vi "Set Magnet Vector Field.vi"(8 "error in (no error)":errorcluster, 9 "Target Rate (T/min)":dbl, 10 "Target Field (T)":dbl[](array[numeric]), 11 "Instrument.VRM in":refnum<class "Instrument.OxfordVRM.lvclass">) -> (0 "error out":errorcluster, 3 "Instrument.VRM out":refnum<class "Instrument.OxfordVRM.lvclass">)   [LabVIEW 2019, in "Instrument.OxfordVRM.lvclass"]
uses:
  Instrument.OxfordVRM.lvclass
  Typedefs/Instrument.VRM.Commands-enum.ctl
  Typedefs/Instrument.VRM.setMagnet-cluster.ctl
  Typedefs/VRM Targets--Cluster.ctl
  Typedefs/VRM Magnet Axis--Enum.ctl
  5e873d59-b7fa-4b76-b36a-7150f831c1b5.vi
  5e873d59-b7fa-4b76-b36a-7150f831c1b5.vi/9026e099-2f45-42fd-b5f2-7045f12962a4.vi
  5e873d59-b7fa-4b76-b36a-7150f831c1b5.vi/9026e099-2f45-42fd-b5f2-7045f12962a4.vi/94005640-8c22-463d-97a2-e8991734048f.vi
  5e873d59-b7fa-4b76-b36a-7150f831c1b5.vi/9026e099-2f45-42fd-b5f2-7045f12962a4.vi/52164787-c95e-474d-af3d-433121107a3c.vi
  5e873d59-b7fa-4b76-b36a-7150f831c1b5.vi/9026e099-2f45-42fd-b5f2-7045f12962a4.vi/52164787-c95e-474d-af3d-433121107a3c.vi/53ccfac9-2453-43af-8059-1cd8c477cd5d.vi
  <userlib>/LevyLab/Levylab Instruments/SMOs/RemoteControl/API/Remote Client.vi
  <vilib>/JDP Science/JSONtext/JSON text to Variant.vi
  <vilib>/JDP Science/JSONtext/LVClass Serializer/JSONtext LVClass Serializer.lvclass
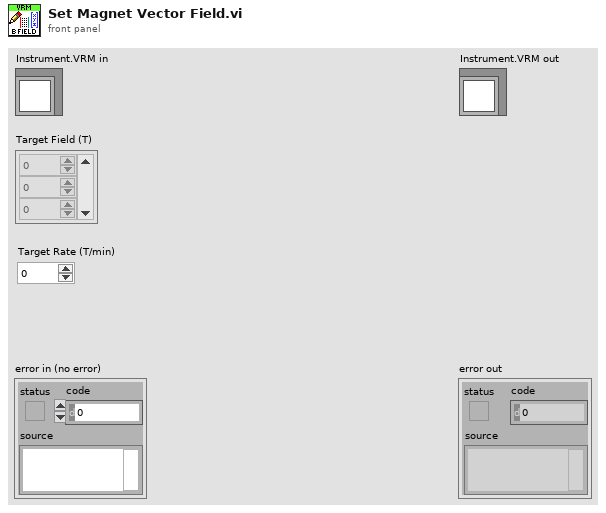
[diagram p1: front panel]
types:
  T1 = typedef "Instrument.OxfordVRM.lvclass/VRM Magnet Axis--Enum.ctl" = enum16{"Z", "X", "Y", "ALL"}
  T2 = typedef "Instrument.OxfordVRM.lvclass/Instrument.VRM.setMagnet-cluster.ctl" = cluster{"Target":T3}
  T3 = typedef "Instrument.OxfordVRM.lvclass/VRM Targets--Cluster.ctl" = cluster{"Field (T)":dbl[], "Field Rate (T/min)":dbl, "Axis":T1}
  T4 = typedef "Instrument.OxfordVRM.lvclass/Instrument.VRM.Commands-enum.ctl" = enum16{"setAction", "setTarget", "setMagnetField", "getStatus", "getTarget", "getMagnetField"}
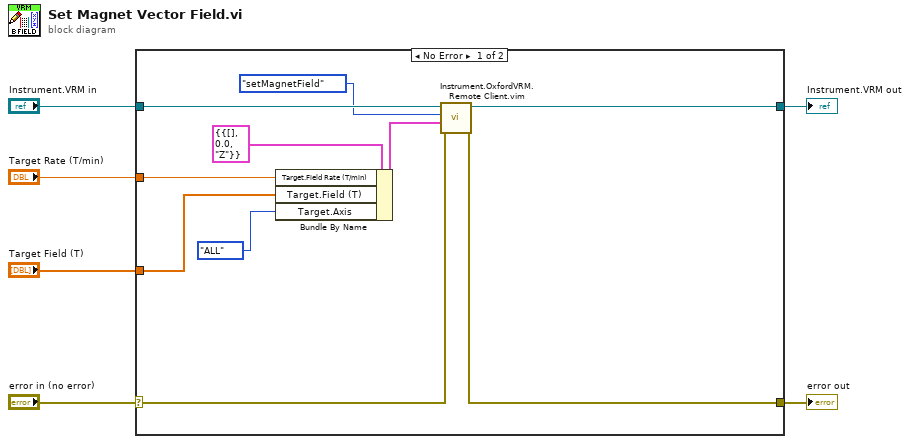
[diagram p0: block diagram]
diagram:
  n1 = case shown="No Error" "error in (no error)" {
    selector: "error in (no error)" -> [w12 w18]
    tunnel: [w8 w18] -> w6
    tunnel: "Instrument.VRM in" -> [w16 w17]
    tunnel: [w15 w17] -> w4
    tunnel: "Target Field (T)" -> [w10 _]
    tunnel: "Target Rate (T/min)" -> [w13 _]
    frame No Error {
      n2 = Bundle By Name(cluster=T2 {"Target"={"Field (T)"=[], "Field Rate (T/min)"=0.0, "Axis"=enum."Z"}} ("output cluster"), "Target.Field Rate (T/min)"=w13, "Target.Field (T)"=w10, "Target.Axis"=VRM_Magnet_Axis--Enum."ALL" ("Axis")) -> (w7:T2)
      n3 = call "Instrument.OxfordVRM.Remote Client.vim"("error in (no error)"=w12, "Data"=w7, "Commands"=Instrument.VRM.Commands-enum."setMagnetField", "Instrument.VRM in"=w16) -> ("error out"=w8:errorcluster, "Instrument.VRM out"=w15:refnum<class "Instrument.OxfordVRM.lvclass">)  [unwired: 5 in, 1 out]
    }
    frame Error {
    }
  }
  "Instrument.VRM out" <- w4
  "error out" <- w6
